vi "ziGetVoltageCalcVec.vi"(8 "Imp50 (F)":bool, 9 "VGain":dbl, 10 "DemodVoltage (Vrms)":cdb[](array[numeric]) format="%#_6p", 11 "Mode":enum16{"From Sig Out", "Signal Input", "HF2CA"}(ring)) -> (2 "Vz (Vrms)":cdb[](array[numeric]) format="%#_6p")   [LabVIEW 2015, in "Zurich Instruments LabOne.lvlib"]
uses:
  Zurich Instruments LabOne.lvlib
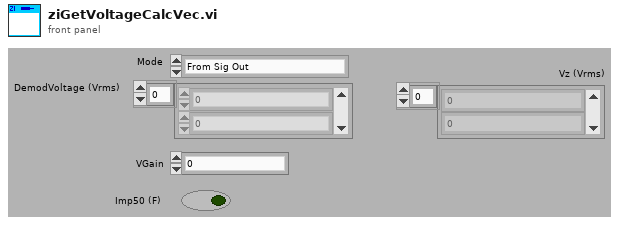
[diagram p1: front panel]
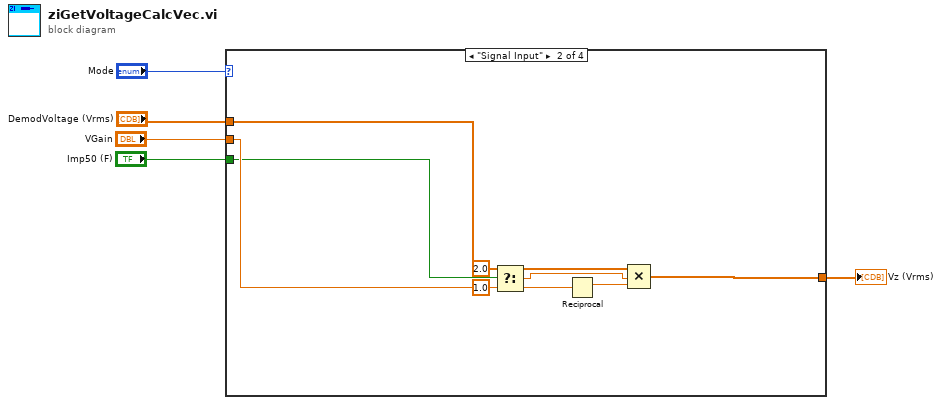
[diagram p0: block diagram]
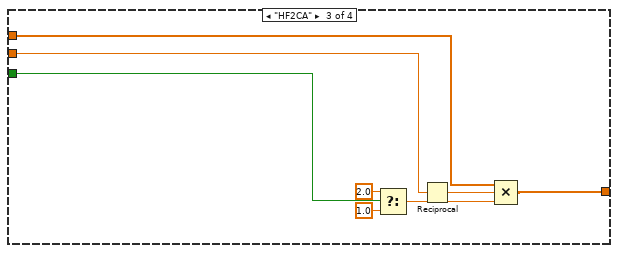
[diagram p3: hidden frame]
diagram:
  n1 = case shown="\"Signal Input\"" "Mode" {
    tunnel: "Imp50 (F)" -> [_ w7 w15 _]
    tunnel: [w6 w13 w17 _] -> w1
    tunnel: "DemodVoltage (Vrms)" -> [w6 w14 w18 _]
    tunnel: "VGain" -> [_ w12 w19 _]
    frame "From Sig Out" {
    }
    frame "Signal Input" {
      n2 = Select(t=2.0, s=w7, f=1.0) -> (s? t:f=w8:dbl)
      n3 = Reciprocal(x=w12) -> (1/x=w9:dbl)
      n4 = Compound Arithmetic op=MULTIPLY(w14, w8, w9) -> (w13:cdb[])
    }
    frame "HF2CA" {
      n5 = Select(t=2.0, s=w15, f=1.0) -> (s? t:f=w20:dbl)
      n6 = Reciprocal(x=w19) -> (1/x=w16:dbl)
      n7 = Compound Arithmetic op=MULTIPLY(w18, w16, w20) -> (w17:cdb[])
    }
    frame Default {
    }
  }
  "Vz (Vrms)" <- w1
